vi "Append Text HF.vi"(0 "PDF Report IN":refnum<class "PDF Report Class.lvclass">, 2 "Header or footer":T1={"Start at page"=1, "Cell Alignment"=4, "Line spacing"=enum."Select", "Text"="", "Font complete"={"Name"="", "Size"=-1.0, "Color"=0, "Style"={"Bold"=FALSE, "Italic"=FALSE, "Underline"=FALSE, "Strikeout"=FALSE}, "Type"={"Type&direction"=enum."Select", "Embedded"=FALSE, "Encoding"=""}}, "Link"=""}, 11 "error in (no error)":errorcluster, 13 "Position":T9) -> (4 "PDF Report OUT":refnum<class "PDF Report Class.lvclass">, 15 "error out":errorcluster)   [LabVIEW 2019]
doc: "Appends <B>text</B> in a column header (or footer). You can use this polymorphic VI to append a colomn to a header (or footer). The data type you wire to the <B>Header or footer</B> input determines the polymorphic instance to use.\n\nThe header (or footer) can be divided up into three columns. Each column has the same width. The number of header (or footer) that you add determines the number of columns.\n\n<B>FRANÇAIS</B>\nAjoute du <B>texte</B> dans une colonne d'un en-tête (ou d'un pied de page). Vous pouvez utiliser ce VI polymorphique pour ajouter une colonne à un en-tête (ou un pied de page). Le type de variable que vous reliez au terminal <B>Header or footer</B> détermine l'instance polymorphique à utiliser.\n\nL'en-tête (ou le pied de page) peut être divisé en un maximum de trois colonnes. Chaque colonne a la même largeur. Le nombre d'en-têtes (ou de pieds de page) que vous ajoutez détermine le nombre de colonnes.\n\n\n\nVersion 1.0\nDeveloped by Jean-Marc Simard\nCopyright © 2012, Exaprom Inc.\nAll rights reserved.\nLicense: BSD\n\nWith iTextSharp 4.1.6 (http://itextsharp.sourceforge.net)\nunder Mozilla Public License Version 1.1\n(http://www.mozilla.org/MPL/MPL-1.1.html)"
uses:
  <userlib>/Exaprom PDF/LV Class/PDF Report Class/PDF Report Class.lvclass
  <userlib>/Exaprom PDF/Controls/Header, Footer and Watermark Controls/Header or Footer.ctl
  <userlib>/Exaprom PDF/Controls/Header, Footer and Watermark Controls/Header or Footer  Text cluster.ctl
  <userlib>/Exaprom PDF/Controls/Table Controls/Cell Alignment 20px.ctl
  <userlib>/Exaprom PDF/Controls/Text Controls/Line spacing.ctl
  <userlib>/Exaprom PDF/Controls/Font Controls/Font complete cluster horizontal.ctl
  <userlib>/Exaprom PDF/Controls/Font Controls/Font size.ctl
  <userlib>/Exaprom PDF/Controls/Font Controls/Font color.ctl
  <userlib>/Exaprom PDF/Controls/Font Controls/Type and encoding.ctl
  <userlib>/Exaprom PDF/Controls/Text Controls/Unicode/Type and run direction.ctl
  <userlib>/Exaprom PDF/LV Class/Header and Footer Class/VIs/Controls/Header Footer cluster V2.ctl
  <userlib>/Exaprom PDF/Controls/Header, Footer and Watermark Controls/Header Footer Type.ctl
  <userlib>/Exaprom PDF/Controls/Header, Footer and Watermark Controls/Header footer horiz alignment.ctl
  <userlib>/Exaprom PDF/Controls/Table Controls/Cell Vertical alignment.ctl
  <userlib>/Exaprom PDF/Controls/Header, Footer and Watermark Controls/Page number.ctl
  <userlib>/Exaprom PDF/Controls/Header, Footer and Watermark Controls/Header Footer Line.ctl
  C:/Program Files/National Instruments/LabVIEW 2019/user.lib/Exaprom PDF/DLL/itextsharp.dll
  DLL/itextsharp.dll
  <userlib>/Exaprom PDF/LV Class/Fonts Class/Font Class.lvclass
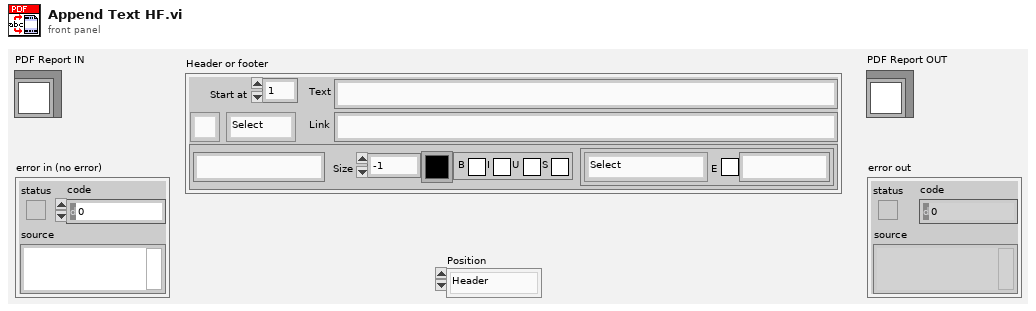
[diagram p1: front panel]
types:
  T1 = typedef "Header or Footer  Text cluster.ctl" = cluster{"Start at page":i32, "Cell Alignment":T2, "Line spacing":T3, "Text":string, "Font complete":T4, "Link":string}
  T2 = typedef "Cell Alignment 20px.ctl" = u16
  T3 = typedef "Line spacing.ctl" = enum16{"Select", "1.0", "1.5", "2.0"}
  T4 = typedef "Font complete cluster horizontal.ctl" = cluster{"Name":string, "Size":T5, "Color":T6, "Style":cluster{"Bold":bool, "Italic":bool, "Underline":bool, "Strikeout":bool}, "Type":T7}
  T5 = typedef "Font size.ctl" = sgl
  T6 = typedef "Font color.ctl" = u32
  T7 = typedef "Type and encoding.ctl" = cluster{"Type&direction":T8, "Embedded":bool, "Encoding":string}
  T8 = typedef "Type and run direction.ctl" = enum16{"Select", "ASCII", "UTF-16", "UTF-16 (default)", "UTF-16 (LTR)", "UTF-16 (RTL)"}
  T9 = typedef "Header or Footer.ctl" = enum16{"Header", "Footer"}
  T10 = typedef "Header Footer cluster V2.ctl" = cluster{"Header or Footer":T9, "Start page":i32, "Start with #":i32, "Type":T11, "Alignment":T12, "Vertical Alignement":T13, "Line spacing":T3, "Image (%)":sgl, "Page #":T14, "Text":string, "Path":string, "Font":T4, "Font refnum":refnum<k24>, "Line":cluster{"Line":T15, "Thickness (points)":sgl, "Colour":T6}, "Vert margin":dbl, "Hyperlink":string}
  T11 = typedef "Header Footer Type.ctl" = enum16{"Select", "Text", "Text + hyperlink", "Page number", "Image", "Image + hyperlink"}
  T12 = typedef "Header footer horiz alignment.ctl" = enum16{"Left", "Center", "Right"}
  T13 = typedef "Cell Vertical alignment.ctl" = enum16{"TOP", "MIDDLE", "BOTTOM"}
  T14 = typedef "Page number.ctl" = cluster{"Text 1":string, "Text 2":string, "Text 3":string}
  T15 = typedef "Header Footer Line.ctl" = enum16{"No line", "Horizontal line"}
  T16 = typedef "Defaut Paragraphe and Line Spacing.ctl" = cluster{" Aligment":T17, "Line spacing":T3}
  T17 = typedef "Texte alignement.ctl" = enum16{"Select", "CENTER", "JUSTIFY", "LEFT", "RIGHT"}
  T18 = typedef "Font complete cluster.ctl" = cluster{"Name":string, "Size":T5, "Color":T6, "Style":cluster{"Bold":bool, "Italic":bool, "Underline":bool, "Strikeout":bool}, "Type":T7}
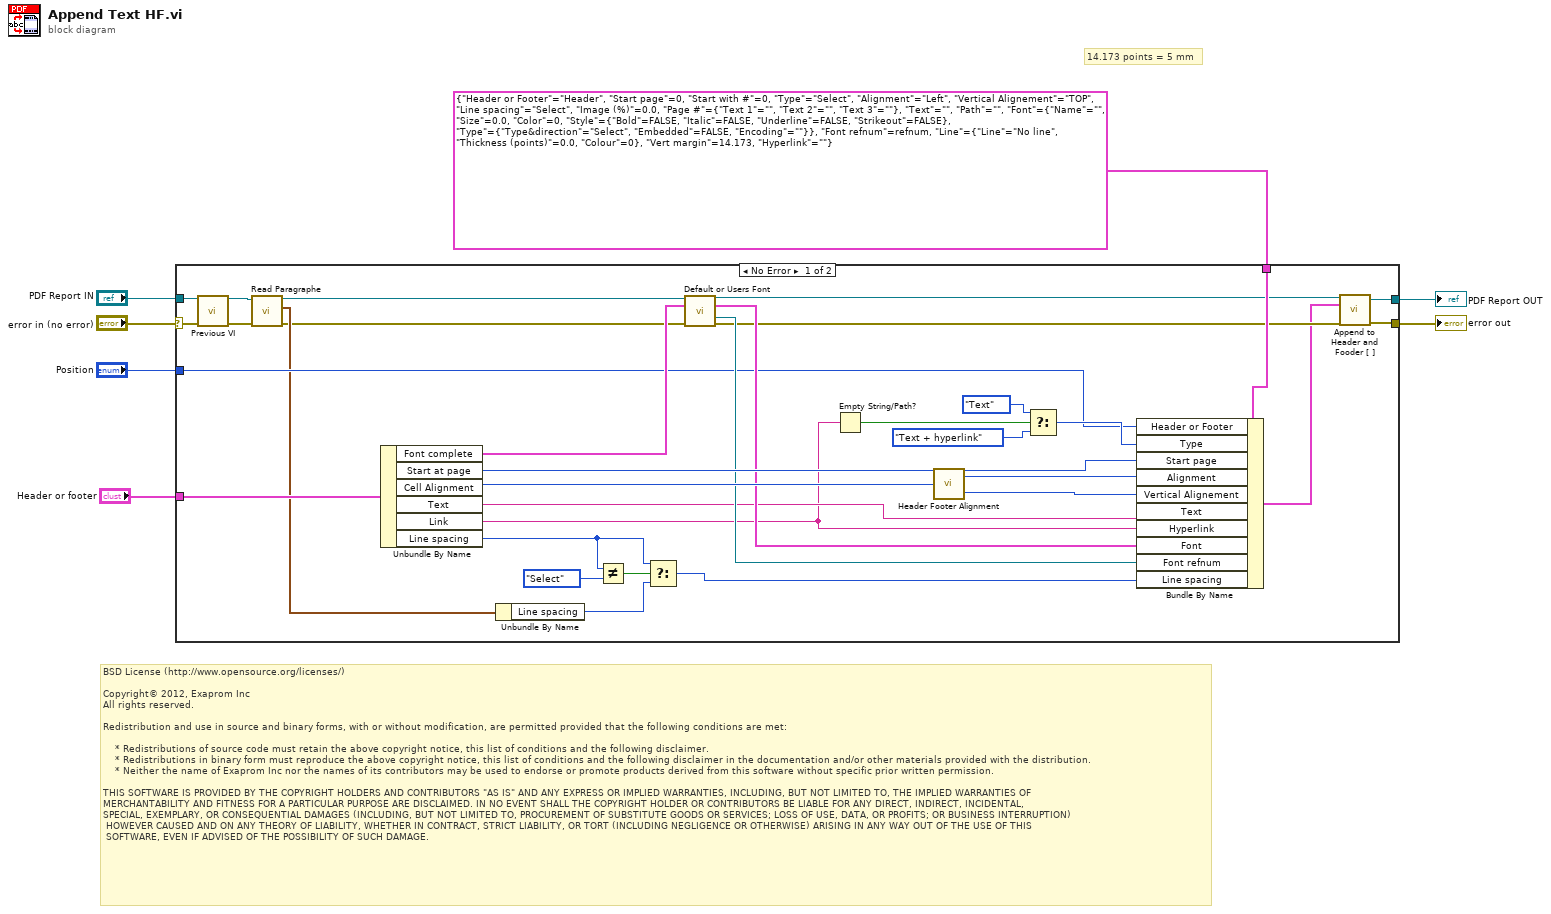
[diagram p0: block diagram]
diagram:
  # "14.173 points = 5 mm"
  # "BSD License (http://www.opensource.org/licenses/)\n\nCopyright© 2012, Exaprom Inc\nAll rights reserved.\n\nRedistribution and use in source and binary forms, with or without modification, are permitted provided that the following conditions are met:\n\n    * Redistributions of source code must retain the above copyright notice, this list of conditions and the following disclaimer.\n    * Redistributions in binary form must reproduce the above copyright notice, this list of conditions and the following disclaimer in the documentation and/or other materials provided with the distribution.\n    * Neither the name of Exaprom Inc nor the names of its contributors may be used to endorse or promote products derived from this software without specific prior written permission.\n\nTHIS SOFTWARE IS PROVIDED BY THE COPYRIGHT HOLDERS AND CONTRIBUTORS \"AS IS\" AND ANY EXPRESS OR IMPLIED WARRANTIES, INCLUDING, BUT NOT LIMITED TO, THE IMPLIED WARRANTIES OF \nMERCHANTABILITY AND FITNESS FOR A PARTICULAR PURPOSE ARE DISCLAIMED. IN NO EVENT SHALL THE COPYRIGHT HOLDER OR CONTRIBUTORS BE LIABLE FOR ANY DIRECT, INDIRECT, INCIDENTAL,\nSPECIAL, EXEMPLARY, OR CONSEQUENTIAL DAMAGES (INCLUDING, BUT NOT LIMITED TO, PROCUREMENT OF SUBSTITUTE GOODS OR SERVICES; LOSS OF USE, DATA, OR PROFITS; OR BUSINESS INTERRUPTION)\n HOWEVER CAUSED AND ON ANY THEORY OF LIABILITY, WHETHER IN CONTRACT, STRICT LIABILITY, OR TORT (INCLUDING NEGLIGENCE OR OTHERWISE) ARISING IN ANY WAY OUT OF THE USE OF THIS\n SOFTWARE, EVEN IF ADVISED OF THE POSSIBILITY OF SUCH DAMAGE."
  n1 = case shown="No Error" "error in (no error)" {
    selector: "error in (no error)" -> [w30 w42]
    tunnel: "PDF Report IN" -> [w31 w41]
    tunnel: "Position" -> [w18 _]
    tunnel: [w25 w41] -> w5
    tunnel: [w24 w42] -> w4
    tunnel: "Header or footer" -> [w29 _]
    tunnel: T10 {"Header or Footer"=enum."Header", "Start page"=0, "Start with #"=0, "Type"=enum."Select", "Alignment"=enum."Left", "Vertical Alignement"=enum."TOP", "Line spacing"=enum."Select", "Image (%)"=0.0, "Page #"={"Text 1"="", "Text 2"="", "Text 3"=""}, "Text"="", "Path"="", "Font"={"Name"="", "Size"=0.0, "Color"=0, "Style"={"Bold"=FALSE, "Italic"=FALSE, "Underline"=FALSE, "Strikeout"=FALSE}, "Type"={"Type&direction"=enum."Select", "Embedded"=FALSE, "Encoding"=""}}, "Font refnum"=refnum, "Line"={"Line"=enum."No line", "Thickness (points)"=0.0, "Colour"=0}, "Vert margin"=14.173, "Hyperlink"=""} ("Cluster") -> [w32 _]
    frame No Error {
      n2 = call <userlib>:"Previous VI.vi"("PDF Report IN"=w31, "error in (no error)"=w30) -> ("PDF Report OUT"=w16:refnum<class "PDF Report Class.lvclass">, "error out"=w17:errorcluster)  [unwired: 12 out]
      n3 = call-dynamic "Read Paragraphe.vi"("error in (no error)"=w17, "PDF Report Class in"=w16) -> ("error out"=w9:errorcluster, "Paragraphe cluster"=w13:T16, "PDF Report Class out"=w8:refnum<class "PDF Report Class.lvclass">)  [unwired: 7 in]
      n4 = Unbundle By Name(w29) -> ("Font complete"=w28:T4, "Start at page"=w36:i32, "Cell Alignment"=w35:T2, "Text"=w20:string, "Link"=w19:string, "Line spacing"=w11:T3)
      n5 = Unbundle By Name(w13) -> ("Line spacing"=w12:T3)
      n6 = Not Equal?(x=w11, y=Line_spacing."Select") -> (x != y?=w14:bool)
      n7 = Select(t=w11, s=w14, f=w12) -> (s? t:f=w10:T3)
      n8 = call <userlib>:"Default or Users Font.vi"("PDF Report"=w8, "Font"=w28, "error in (no error)"=w9) -> ("PDF Report duplicate"=w23:refnum<class "PDF Report Class.lvclass">, "Font OUT"=w27:T18, "Font Ref"=w26:refnum<k24>, "error out"=w22:errorcluster)  [unwired: 7 in, 2 out]
      n9 = Empty String/Path?(string/path=w19) -> (empty?=w40:bool)
      n10 = call <userlib>:"Header Footer Alignment.vi"("Cell Alignment"=w35) -> ("Vertical Alignement"=w33:T13, "Horizontal Alignment"=w34:T12)  [unwired: 2 out]
      n11 = Select(t=Header_Footer_Type."Text" ("Type"), s=w40, f=Header_Footer_Type."Text + hyperlink" ("Type")) -> (s? t:f=w39:T11)
      n12 = Bundle By Name(cluster=w32, "Header or Footer"=w18, "Type"=w39, "Start page"=w36, "Alignment"=w34, "Vertical Alignement"=w33, "Text"=w20, "Hyperlink"=w19, "Font"=w27, "Font refnum"=w26, "Line spacing"=w10) -> (w21:T10)
      n13 = call <userlib>:"Append to Header and Fooder [ ].vi"("PDF Report IN"=w23, "Header and Footer"=w21, "error in (no error)"=w22) -> ("PDF Report OUT"=w25:refnum<class "PDF Report Class.lvclass">, "error out"=w24:errorcluster)  [unwired: 11 in]
    }
    frame Error {
    }
  }
  "PDF Report OUT" <- w5
  "error out" <- w4
